vi "Multiply Force.vi"(10 "force in":dbl, 11 "Mallet in":refnum<class "Mallet.lvclass">) -> (2 "force out":dbl)   [LabVIEW 2023, in "Mallet.lvclass"]
uses:
  Mallet.lvclass
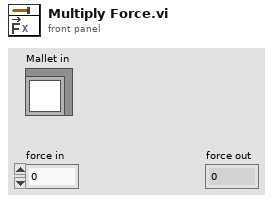
[diagram p1: front panel]
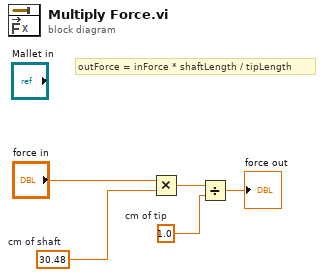
[diagram p0: block diagram]
diagram:
  w2 = 30.48  # cm of shaft
  w4 = 1.0  # cm of tip
  # "outForce = inForce * shaftLength / tipLength"
  n1 = Multiply(x="force in", y=w2) -> (x*y=w5:dbl)
  n2 = Divide(x=w5, y=w4) -> (x/y=→"force out":dbl)
